vi "wrap-array.vi"(1 "Array In":dbl[](array[numeric])) -> (0 "Array Out":dbl[](array[numeric]))   [LabVIEW 2021]
doc: "This VI Wraps phase data to stay between 180 and -180 degrees."
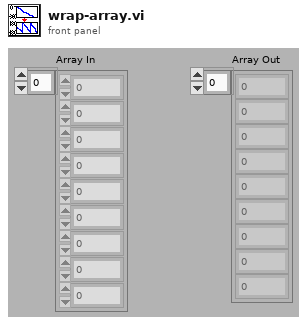
[diagram p1: front panel]
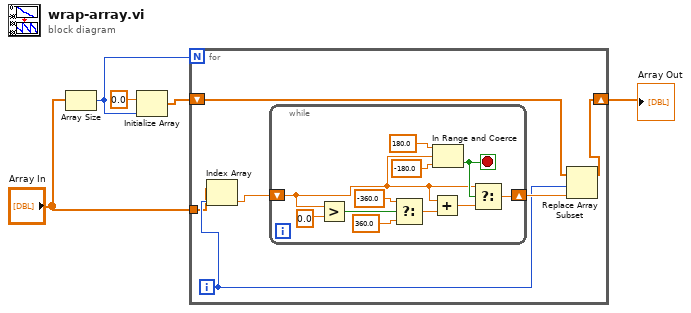
[diagram p0: block diagram]
diagram:
  n1 = Array Size(array="Array In") -> (size(s)=w5:i32)
  n2 = Initialize Array(0.0 ("element"), w5) -> (w3:dbl[])
  n3 = for {
    N: w5 -> [_]
    shift-right: [w9] -> w2
    shift-left: w3 -> [w10]
    tunnel: "Array In" -> [w7]
    i -> [w8]
    n4 = Index Array(array=w7, index=w8) -> (element=w6:dbl)
    n5 = while {
      shift-right: [w12] -> w11
      shift-left: w6 -> [w14]
      stop <- w15 stop-if-true
      n6 = Greater?(x=w14, y=0.0) -> (0:w21:bool)
      n7 = Select(t=-360.0, s=w21, f=360.0) -> (s? t:f=w18:dbl)
      n8 = Add(x=w14, y=w18) -> (x+y=w13:dbl)
      n9 = In Range and Coerce(upper limit=180.0, x=w14, lower limit=-180.0) -> (In Range?=w15:bool)  [unwired: 1 out]
      n10 = Select(t=w14, s=w15, f=w13) -> (s? t:f=w12:dbl)
    }
    n11 = Replace Array Subset(array=w10, new element=w11, index=w8) -> (w9:dbl[])
  }
  "Array Out" <- w2
